vi "test_ThreeSessThreePinTwoInstrTwoSiteReservation_CallGetConnectionsFromPinsForOneDcPowerPinAllSites_ReturnsTwoConnections.vi"(8 "error in":errorcluster) -> (0 "error out":errorcluster, 2 "result":string, 3 "pass":bool)   [LabVIEW 2020, in "MeasurementServerTests.lvlib"]
uses:
  MeasurementServerTests.lvlib
  Runtime/MeasurementLink Session Management/Session Reservation/Connection.ctl
  Runtime/MeasurementLink Session Management/Session Reservation/Session Reservation.lvclass
  Runtime/MeasurementLink Session Management/Session Reservation/Connection with Session.ctl
  b3e5c3be-b7a7-4b6e-86ee-709eea9cb752.vi
  c3cb69a0-23cd-49fc-99d1-8c54773f0200.vi
  75c1e948-44f8-456a-9c7f-fb5b0af28fdb.vi
  66557e30-f4e9-402c-98cb-662df6234d12.vi
  Runtime/MeasurementLink niDCPower/Instrument/Instrument.lvclass
  Runtime/MeasurementLink Session Management/Session Reservation/Pin Type.ctl
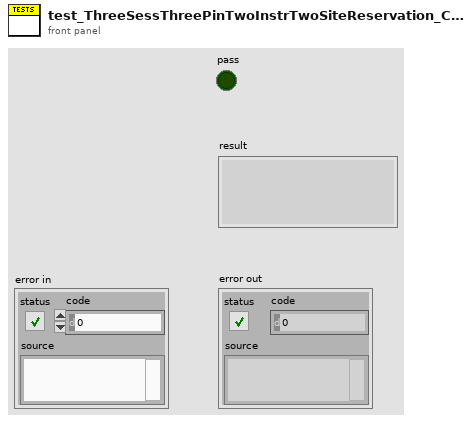
[diagram p1: front panel]
types:
  T1 = typedef "MeasurementLink Session Management.lvlib/Session Reservation.lvclass/Pin Type.ctl" = enum16{"All Pins", "DUT Pins", "System Pins"}
  T2 = typedef "MeasurementLink Session Management.lvlib/Session Reservation.lvclass/Connection.ctl" = cluster{"pin or relay name":string, "site":i32, "instrument type id":string, "channel":string}
  T3 = typedef "MeasurementLink Session Management.lvlib/Session Reservation.lvclass/Connection with Session.ctl" = cluster{"connection":T2, "session":variant}
  T4 = typedef "MeasurementLink Session Management.lvlib/Session Reservation.lvclass/Data.ctl" = cluster{"session and driver infos":T5[], "pin or relay names":string[], "connection map":refnum<class "Connection Map.lvclass">, "pin map context":T9, "reservation observer":refnum<class "IReservationObserver.lvclass">, "dvr valid":bool}
  T5 = typedef "MeasurementLink Session Management.lvlib/Session Reservation.lvclass/Session and Driver Info.ctl" = cluster{"session info":T6, "session":variant, "instrument":refnum<class "IInstrument.lvclass">}
  T6 = typedef "MeasurementLink Session Management Client.lvlib/ni_measurementlink_sessionmanagement_v1_SessionInformation.ctl" = cluster{"session":T7, "resource_name":string, "channel_list":string, "instrument_type_id":string, "session_exists":bool, "channel_mappings":T8[]}
  T7 = typedef "MeasurementLink Session Management Client.lvlib/nidevice_grpc_Session.ctl" = cluster{"name":string}
  T8 = typedef "MeasurementLink Session Management Client.lvlib/ni_measurementlink_sessionmanagement_v1_ChannelMapping.ctl" = cluster{"pin_or_relay_name":string, "site":i32, "channel":string}
  T9 = typedef "MeasurementLink Session Management Client.lvlib/ni_measurementlink_PinMapContext.ctl" = cluster{"pin_map_id":string, "sites":i32[]}
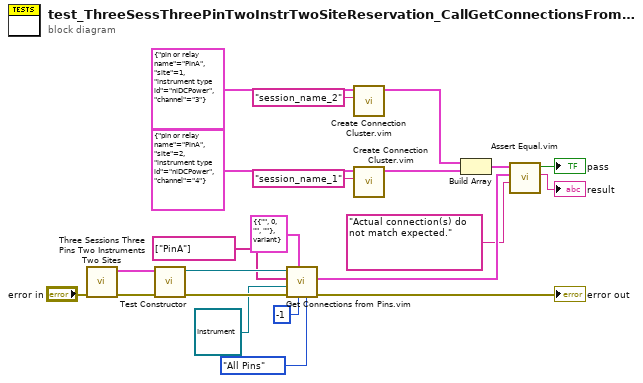
[diagram p0: block diagram]
diagram:
  n1 = call "Three Sessions Three Pins Two Instruments Two Sites.vi"("error in"="error in") -> ("error out"=w12:errorcluster, "data out"=w11:T4)  [unwired: 9 in]
  n2 = call "Test Constructor.vi"("error in"=w12, "data"=w11) -> ("error out"=w21:errorcluster, "Session Reservation out"=w20:refnum<class "Session Reservation.lvclass">)  [unwired: 8 in]
  n3 = call "Get Connections from Pins.vim"("pin type"=Pin_Type."All Pins", "site"=-1, "connection type"=T3 {"connection"={"pin or relay name"="", "site"=0, "instrument type id"="", "channel"=""}, "session"=variant} ("connection"), "error in"=w21, "instrument"=refnum<class "Instrument.lvclass"> refnum ("MeasurementLink niDCPower.lvlib:Instrument.lvclass"), "pin or relay names"=string[] ["PinA"], "session reservation in"=w20) -> ("error out"=→"error out":errorcluster, "connections"=w17:T3[])  [unwired: 2 in, 1 out]
  n4 = call "Create Connection Cluster.vim"("session in"="session_name_2", "hardware independent connection in"=T2 {"pin or relay name"="PinA", "site"=1, "instrument type id"="niDCPower", "channel"="3"} ("connection")) -> ("connection out"=w10:T3)  [unwired: 9 in]
  n5 = call "Create Connection Cluster.vim"("session in"="session_name_1", "hardware independent connection in"=T2 {"pin or relay name"="PinA", "site"=2, "instrument type id"="niDCPower", "channel"="4"} ("connection")) -> ("connection out"=w9:T3)  [unwired: 9 in]
  n6 = Build Array(w10, w9) -> (w8:T3[])
  n7 = call "Assert Equal.vim"("failure message"="Actual connection(s) do not match expected.", "actual value"=w17, "expected value"=w8) -> ("message"=→"result":string, "equal?"=→"pass":bool)  [unwired: 7 in]
